vi "Looking.vi"(5 "Break Timeout (ms)":dbl=50.0, 7 "Fixation Radius (px)":dbl, 10 "Desired Position":cluster{"X":dbl, "Y":dbl}, 11 "Eye Position":cluster{"X":dbl, "Y":dbl}) -> (2 "Looking Unfiltered":bool, 3 "Looking":bool)   [LabVIEW 2014, in "BehaviorData.lvclass"]
doc: "Determine if the subject is looking at a location (Desired Position input) within a certain radius. It will output this on Looking Unfiltered. In addition it can require the test subject break fixation for a certain time (Break Timeouts) and output that on Looking."
uses:
  BehaviorData.lvclass
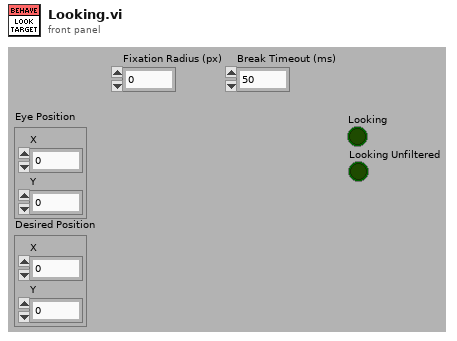
[diagram p1: front panel]
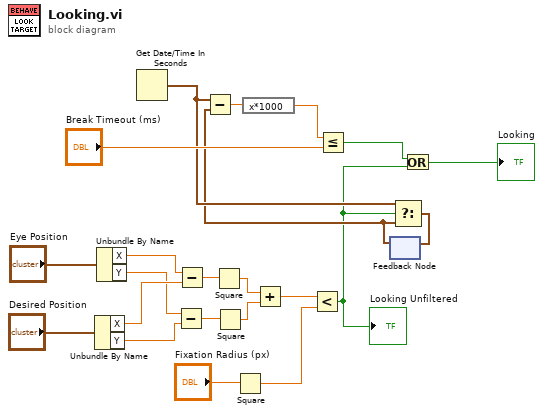
[diagram p0: block diagram]
diagram:
  n1 = Unbundle By Name("Desired Position") -> ("X"=w19:dbl, "Y"=w18:dbl)
  n2 = Unbundle By Name("Eye Position") -> ("X"=w20:dbl, "Y"=w17:dbl)
  n3 = Get Date/Time In Seconds() -> (seconds since 1Jan1904=w7:timestamp)
  n4 = Subtract(x=w17, y=w18) -> (x-y=w15:dbl)
  n5 = Subtract(x=w20, y=w19) -> (x-y=w16:dbl)
  n6 = Square(x=w16) -> (x^2=w14:dbl)
  n7 = Square(x=w15) -> (x^2=w13:dbl)
  n8 = Square(x="Fixation Radius (px)") -> (x^2=w2:dbl)
  n9 = Add(x=w14, y=w13) -> (x+y=w12:dbl)
  n10 = Less?(x=w12, y=w2) -> (x < y?=w4:bool)
  "Looking Unfiltered" <- w4
  n11 = feedback #1() -> (w5:timestamp)  [unwired: 1 in]
  n12 = Subtract(x=w7, y=w5) -> (x-y=w11:dbl)
  n13 = expression code="x*1000"(w11) -> (w10:dbl)
  n14 = Less Or Equal?(x=w10, y="Break Timeout (ms)") -> (x <= y?=w8:bool)
  n15 = Select(t=w7, s=w4, f=w5) -> (s? t:f=w6:timestamp)
  n16 = feedback-in #1(w6) -> ()
  n17 = Or(x=w8, y=w4) -> (x .or. y?=→"Looking":bool)
